vi "open with serial number.vi"(8 "error in (no error)":errorcluster, 11 "serial_number":string="Z8KHE") -> (0 "error out":errorcluster, 3 "Relay Identifier":i32=355835048)   [LabVIEW 2022 SP3, in "usb_relay_device.lvlib"]
doc: "int EXPORT_API usb_relay_device_open_with_serial_number(const char *serial_number, unsigned len);"
uses:
  usb_relay_device.lvlib
  D:/LabVIEWSuite_64_OS/ScanningControl/Switch Modules/RiversideUSBRealy/usb_relay_device.dll
panel:
  in  "len":u32=1
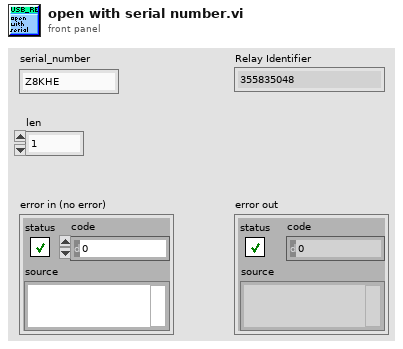
[diagram p1: front panel]
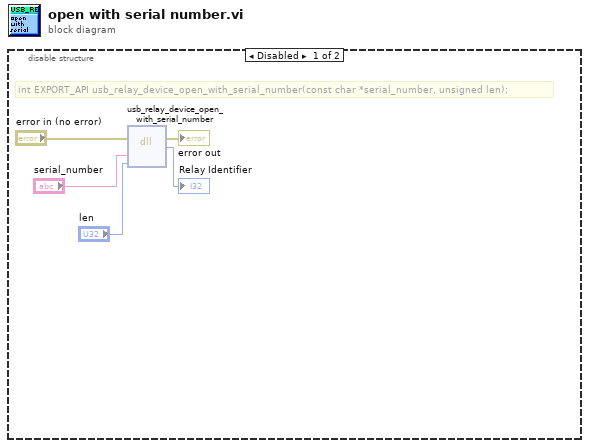
[diagram p0: block diagram]
diagram:
  n1 = disable-structure shown="Disabled" {
    frame Disabled {
      # "int EXPORT_API usb_relay_device_open_with_serial_number(const char *serial_number, unsigned len);"
      n2 = dll-call lib="D:/LabVIEWSuite_64_OS/ScanningControl/Switch Modules/RiversideUSBRealy/usb_relay_device.*" fn="usb_relay_device_open_with_serial_number"(error in="error in (no error)", "serial_number"="serial_number", "len"="len") -> (error out=→"error out":errorcluster, →"Relay Identifier":i32)  [unwired: 4 in, 1 out]
    }
    frame Enabled {
    }
  }
